vi "Scope Read Wfm.vi"(8 "error in (no error)":errorcluster, 10 "TimeOut":u32=5000, 11 "Actor_Scope in":refnum<class "Actor_Scope.lvclass">) -> (0 "error out":errorcluster, 3 "Actor_Scope out":refnum<class "Actor_Scope.lvclass">)   [LabVIEW 2020, in "Actor_Scope.lvlib" / "Actor_Scope.lvclass"]
uses:
  Actor_Scope.lvclass
  C:/Program Files/National Instruments/LabVIEW 2020/vi.lib/ActorFramework/Actor/Actor.lvclass
  Scope_Event.ctl
  <vilib>/ActorFramework/Actor/Actor.lvclass/Actor.ctl
  Actor_Scope.lvclass/Actor_Scope.ctl
  <instrlib>/Agilent 8000 Series/Public/Data/Low Level/Fetch (Waveform).vi
  <instrlib>/Agilent 8000 Series/Agilent 8000 Series.lvlib
  <vilib>/ActorFramework/Actor/Actor.lvclass
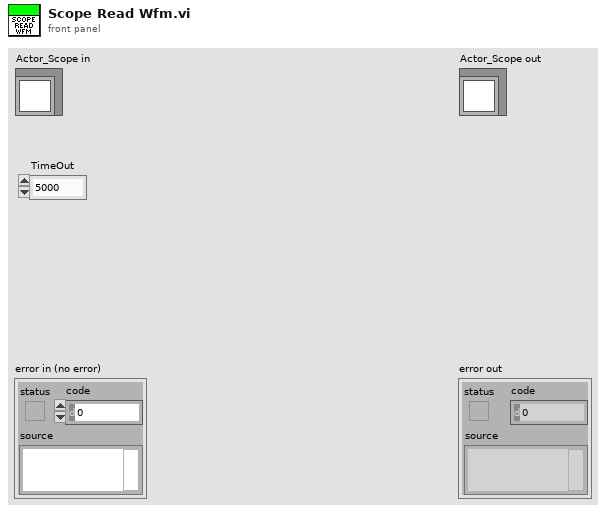
[diagram p1: front panel]
types:
  T1 = typedef "Actor_Scope.lvlib/Actor_Scope.lvclass/Scope_Event.ctl" = enum16{"General Event", "Inited", "Error", "Wfm Acq Complete"}
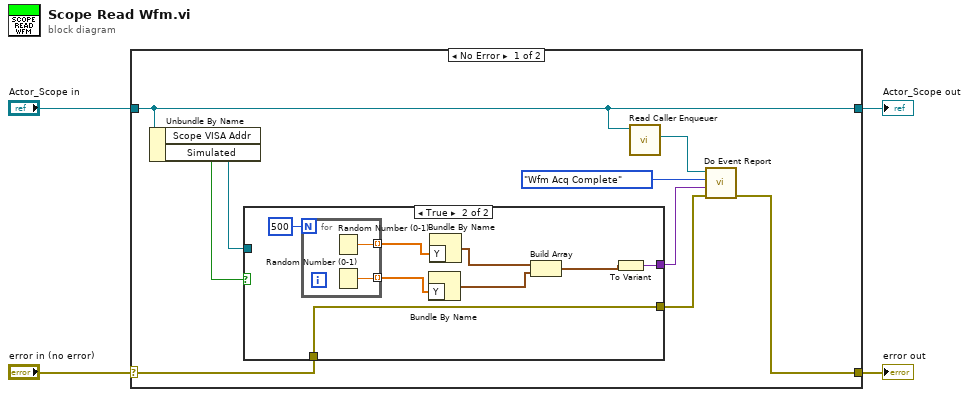
[diagram p0: block diagram]
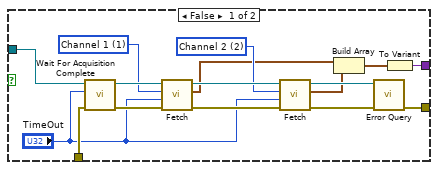
[diagram p2: hidden frame]
diagram:
  n1 = case shown="No Error" "error in (no error)" {
    selector: "error in (no error)" -> [w12 w41]
    tunnel: [w6 w41] -> w3
    tunnel: [w10 w40] -> w1
    tunnel: "Actor_Scope in" -> [w10 w40]
    frame No Error {
      n2 = Unbundle By Name(w10) -> ("Scope VISA Addr"=w13:refnum<visa-resource-name>, "Simulated"=w5:bool)
      n3 = case shown="True" w5 {
        tunnel: w13 -> [w29 _]
        tunnel: w12 -> [w28 w37]
        tunnel: [w24 w37] -> w8
        tunnel: [w23 w36] -> w7
        frame False {
          w20 = 2 items=["Channel 1"=1, "Channel 2"=2, "Channel 3"=3, "Channel 4"=4, "Function 1"=5, "Function 2"=6, "Function 3"=7, "Function 4"=8, "Memory 1"=9, "Memory 2"=10, "Memory 3"=11, "Memory 4"=12] ("Channel (1: Channel 1)")
          w26 = 1 items=["Channel 1"=1, "Channel 2"=2, "Channel 3"=3, "Channel 4"=4, "Function 1"=5, "Function 2"=6, "Function 3"=7, "Function 4"=8, "Memory 1"=9, "Memory 2"=10, "Memory 3"=11, "Memory 4"=12] ("Channel (1: Channel 1)")
          n4 = call <instrlib>:"Wait For Acquisition Complete.vi"("error in (no error)"=w28, "Maximum Time (10000ms)"="TimeOut", "VISA resource name"=w29) -> ("error out"=w25:errorcluster, "VISA resource name out"=w27:refnum<visa-resource-name>)  [unwired: 7 in]
          n5 = call-poly <instrlib>:"Fetch.vi"("error in (no error)"=w25, "Maximum Time (10000ms)"="TimeOut", "Channel (1: Channel 1)"=w26, "VISA resource name"=w27) -> ("error out"=w21:errorcluster, "Waveform Data"=w15:waveform(dbl), "VISA resource name out"=w22:refnum<visa-resource-name>)  [unwired: 5 in]
          n6 = call-poly <instrlib>:"Fetch.vi"("error in (no error)"=w21, "Maximum Time (10000ms)"="TimeOut", "Channel (1: Channel 1)"=w20, "VISA resource name"=w22) -> ("error out"=w17:errorcluster, "Waveform Data"=w16:waveform(dbl), "VISA resource name out"=w18:refnum<visa-resource-name>)  [unwired: 5 in]
          n7 = Build Array(w15, w16) -> (w14:waveform(dbl)[])
          n8 = call <instrlib>:"Error Query.vi"("error in (no error)"=w17, "VISA resource name"=w18) -> ("error out"=w24:errorcluster)  [unwired: 6 in, 3 out]
          n9 = To Variant(anything=w14) -> (Variant=w23:variant)
        }
        frame True {
          n10 = for {
            N: 500 -> [_]
            tunnel: [w39] -> w35 mode=indexing
            tunnel: [w38] -> w34 mode=indexing
            n11 = Random Number (0-1)() -> (number: 0 to 1=w39:dbl)
            n12 = Random Number (0-1)() -> (number: 0 to 1=w38:dbl)
          }
          n13 = Bundle By Name("Y"=w34) -> (w30:waveform(dbl))  [unwired: 1 in]
          n14 = Bundle By Name("Y"=w35) -> (w31:waveform(dbl))  [unwired: 1 in]
          n15 = Build Array(w31, w30) -> (w32:waveform(dbl)[])
          n16 = To Variant(anything=w32) -> (Variant=w36:variant)
        }
      }
      n17 = call <vilib>:"Read Caller Enqueuer.vi"("Actor"=w10) -> ("Caller Enqueuer"=w9:refnum<class "Message Enqueuer.lvclass">)  [unwired: 10 in]
      n18 = call "Do Event Report.vi"("error in (no error)"=w8, "Event Data"=w7, "Scope Events"=Scope_Event."Wfm Acq Complete", "Caller Enqueuer"=w9) -> ("error out"=w6:errorcluster)  [unwired: 6 in, 1 out]
    }
    frame Error {
    }
  }
  "error out" <- w3
  "Actor_Scope out" <- w1
